vi "Linux Get Time Performance Test.vi"() -> ()   [LabVIEW 2021]
uses:
  <vilib>/Platform/TimedLoop/XDataNode/timing_clust.ctl
  <vilib>/Platform/TimedLoop/XDataNode/nitl_modes.ctl
  <vilib>/Platform/TimedLoop/XDataNode/wakeup.ctl
  <vilib>/Platform/TimedLoop/XDataNode/XDataNode.xnode
  <vilib>/Platform/TimedLoop/XDataNode/XDNodeRunTimeDep.lvlib
  Time_CIF_U.lvlib
panel:
  out "avg Linux Time":dbl
  out "max Linux Time":dbl
  out "avg LV Time":dbl
  out "max LV Time":dbl
  out "pass":bool
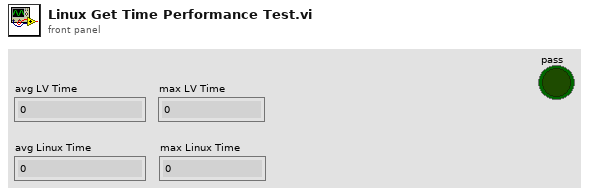
[diagram p1: front panel]
types:
  T1 = typedef "XDNodeRunTimeDep.lvlib/timing_clust.ctl" = cluster{"Expected End [f-1]":u64, "Actual End [f-1]":u64, "Finished Late? [f-1]":bool, "Expected End [i-1]":u64, "Actual End [i-1]":u64, "Finished Late? [i-1]":bool, "Expected Start [i]":u64, "Actual Start [i]":u64, "Expected Start [f]":u64, "Actual Start [f]":u64, "Source Name":string, "Structure Name":string, "Period":i64, "Deadline":i64, "Offset":i64, "Start":i64, "Priority":i32, "Timeout":i32, "Mode":T2, "Wakeup Reason":T3, "Error":errorcluster, "Source Type":string, "Secondary Source Type":string, "Global End Time":u64, "Global Start Time":u64, "Frame Duration":u64, "Iteration Duration":u64, "Assigned CPU":i32, "I/O Scan Engine Mode":u32}
  T2 = typedef "XDNodeRunTimeDep.lvlib/nitl_modes.ctl" = enum32{"No Change", "Process missed periods, maintain original phase", "Discard missed periods, maintain original phase", "Process missed periods, ignore original phase", "Discard missed periods, ignore original phase"}
  T3 = typedef "XDNodeRunTimeDep.lvlib/wakeup.ctl" = enum32{"Normal", "Aborted", "Asynchronous wakeup", "Timing source error", "Timed loop error", "Timeout"}
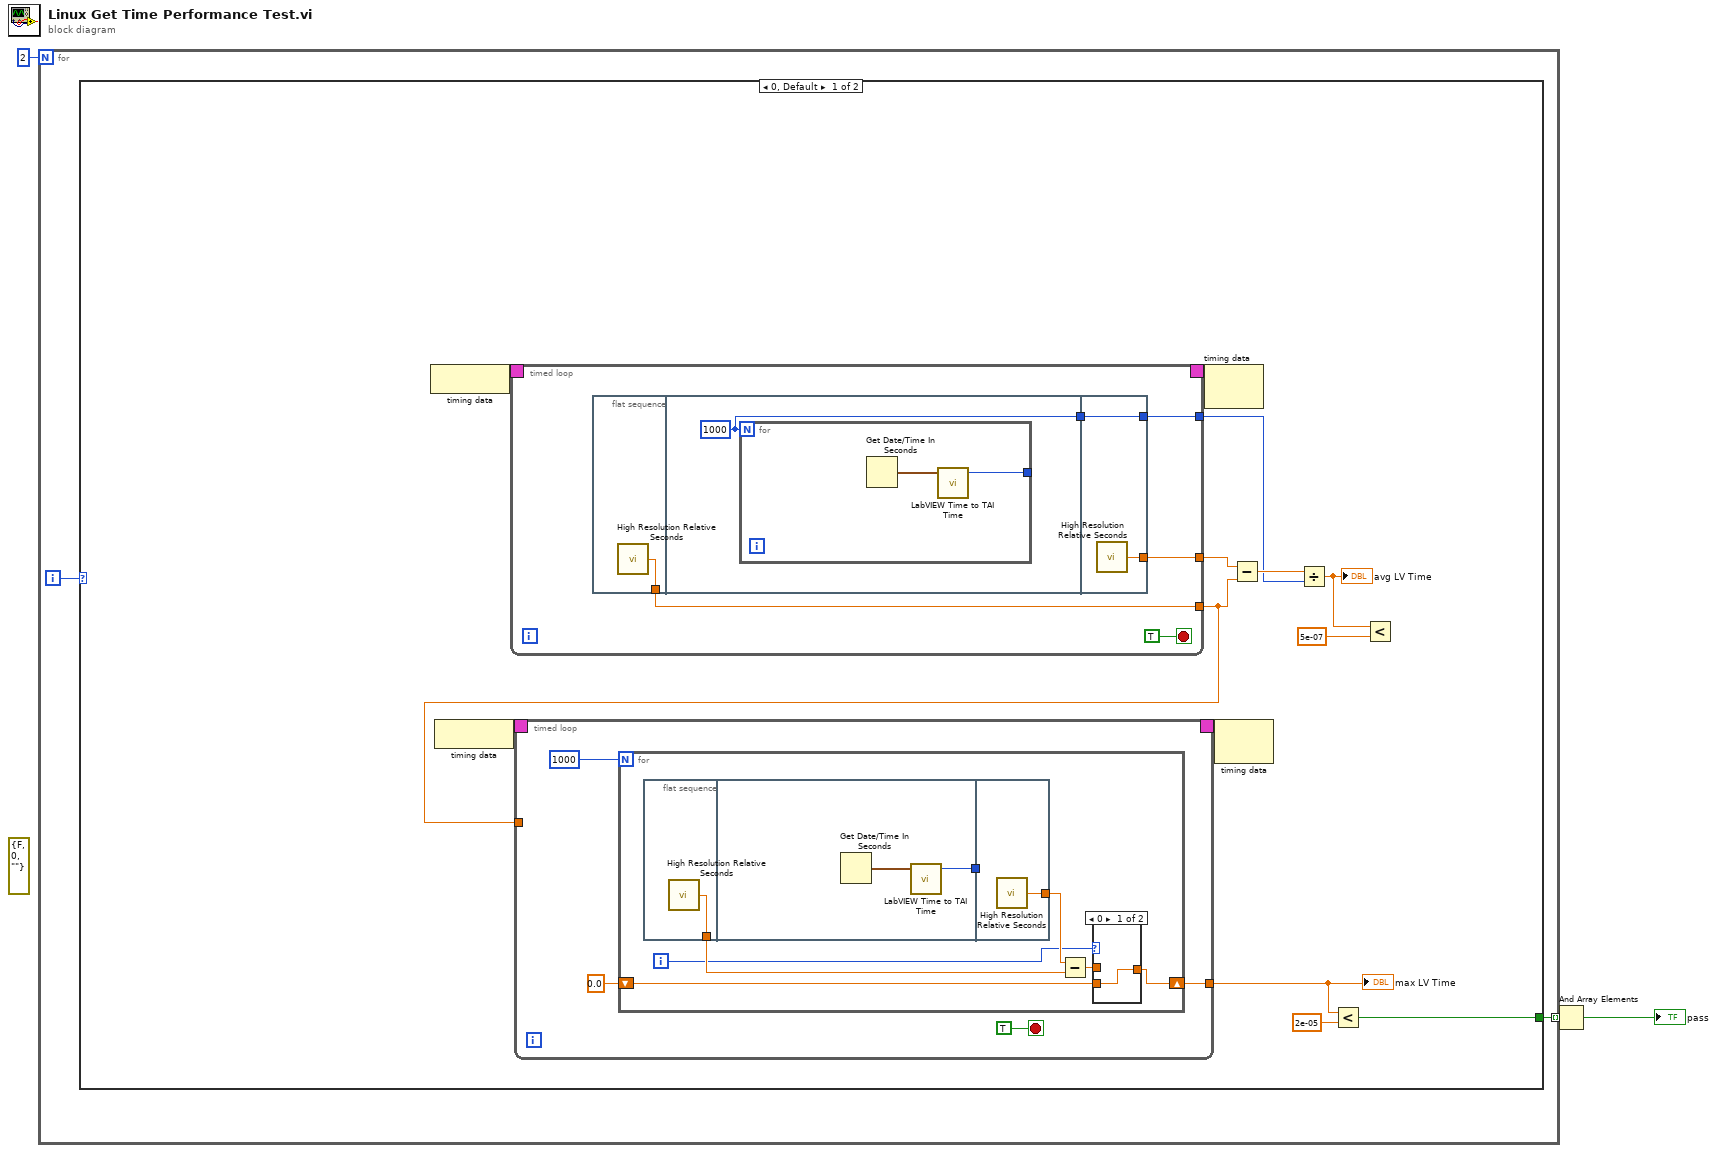
[diagram p0: block diagram]
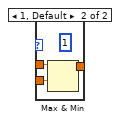
[diagram p2: hidden frame]
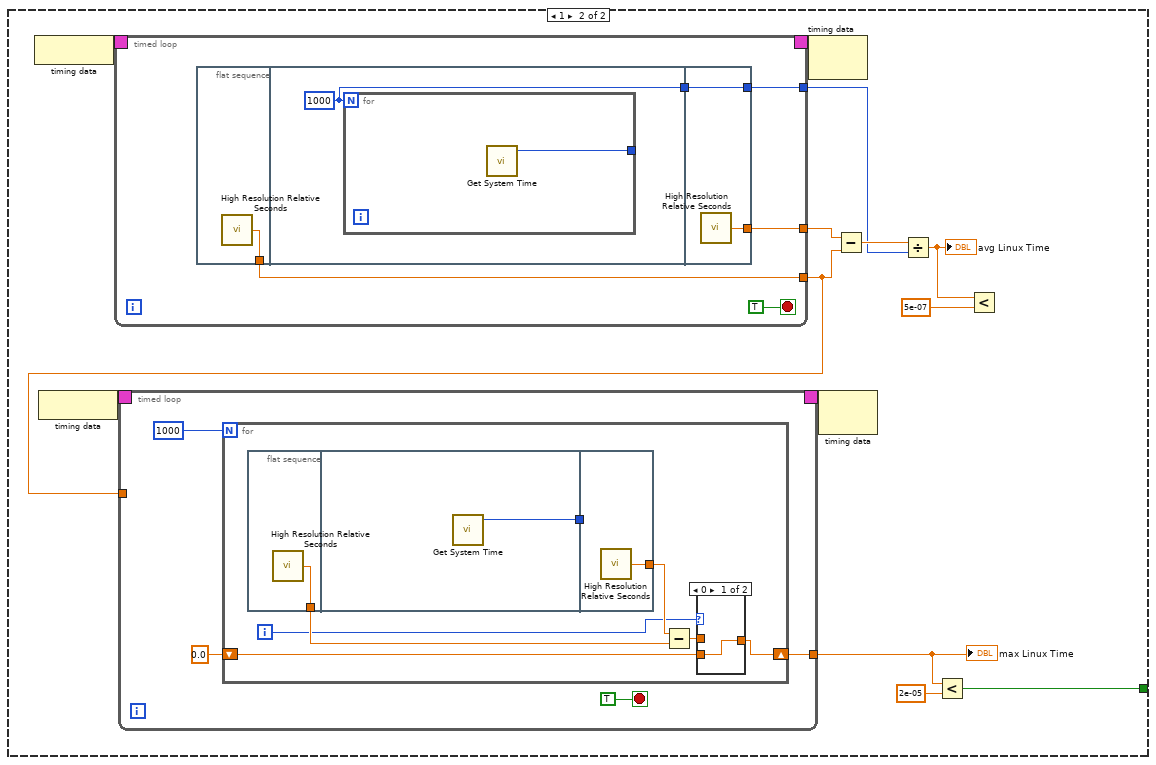
[diagram p3: hidden frame]
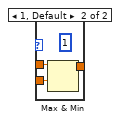
[diagram p4: hidden frame]
diagram:
  (unwired) errorcluster {"status"=FALSE, "code"=0, "source"=""} ("error out")
  n1 = for {
    N: 2 -> [_]
    tunnel: [w5] -> w2 mode=indexing
    i -> [w4]
    n2 = case shown="0, Default" w4 {
      tunnel: [w7 w58] -> w5
      frame 0, Default {
        n3 = node-c288() -> (w18:T1)
        n4 = node-c288() -> (w16:T1)
        n5 = timed-loop {
          timing: w18 -> [_]
          timing-out: [_] -> w17
          tunnel: [w45] -> w14
          tunnel: [w44] -> w6
          tunnel: [w43] -> w12
          stop <- TRUE stop-if-true
          n6 = flat-sequence {
            tunnel: [w47] -> w44
            tunnel: [w48] -> w42
            tunnel: [w52] -> w45
            tunnel: [w51] -> w43
            tunnel: w42 -> [w51]
            frame #0 {
              n7 = call <vilib>:"High Resolution Relative Seconds.vi"() -> ("relative seconds"=w47:dbl)
            }
            frame #1 {
              w48 = 1000
              n8 = for {
                N: w48 -> [_]
                tunnel: [w49] -> _
                n9 = Get Date/Time In Seconds() -> (seconds since 1Jan1904=w50:timestamp)
                n10 = call "LabVIEW Time to TAI Time.vi"("LabVIEW Time (s)"=w50) -> ("TAI Time (ns)"=w49:i64)  [unwired: 4 in]
              }
            }
            frame #2 {
              n11 = call <vilib>:"High Resolution Relative Seconds.vi"() -> ("relative seconds"=w52:dbl)
            }
          }
        }
        n12 = timed-loop {
          timing: w16 -> [_]
          timing-out: [_] -> w15
          tunnel: [w19] -> w9
          tunnel: w6 -> [_]
          stop <- TRUE stop-if-true
          n13 = for {
            N: 1000 -> [_]
            shift-right: [w25] -> w19
            shift-left: 0.0 -> [w26]
            i -> [w24]
            n14 = flat-sequence {
              tunnel: [w34] -> w28
              tunnel: [w35] -> w23
              tunnel: [w37] -> w29
              tunnel: w23 -> [_]
              frame #0 {
                n15 = call <vilib>:"High Resolution Relative Seconds.vi"() -> ("relative seconds"=w34:dbl)
              }
              frame #1 {
                n16 = Get Date/Time In Seconds() -> (seconds since 1Jan1904=w36:timestamp)
                n17 = call "LabVIEW Time to TAI Time.vi"("LabVIEW Time (s)"=w36) -> ("TAI Time (ns)"=w35:i64)  [unwired: 4 in]
              }
              frame #2 {
                n18 = call <vilib>:"High Resolution Relative Seconds.vi"() -> ("relative seconds"=w37:dbl)
              }
            }
            n19 = Subtract(x=w29, y=w28) -> (x-y=w27:dbl)
            n20 = case shown="0" w24 {
              tunnel: w27 -> [_ w33]
              tunnel: w26 -> [w30 w32]
              tunnel: [w30 w31] -> w25
              frame 0 {
              }
              frame 1, Default {
                (unwired) u32 1 ("milliseconds to wait")
                n21 = Max & Min(x=w33, y=w32) -> (max(x,y)=w31:dbl)  [unwired: 1 out]
              }
            }
          }
        }
        "max LV Time" <- w9
        n22 = node-c288(w17) -> ()  [unwired: 1 out]
        n23 = node-c288(w15) -> ()  [unwired: 1 out]
        n24 = Subtract(x=w14, y=w6) -> (x-y=w13:dbl)
        n25 = Divide(x=w13, y=w12) -> (x/y=w11:dbl)
        "avg LV Time" <- w11
        n26 = Less?(x=w9, y=2e-05) -> (x < y?=w7:bool)
        n27 = Less?(x=w11, y=5e-07) -> ()  [unwired: 1 out]
      }
      frame 1 {
        n28 = node-c288() -> (w69:T1)
        n29 = node-c288() -> (w67:T1)
        n30 = timed-loop {
          timing: w69 -> [_]
          timing-out: [_] -> w68
          tunnel: [w95] -> w65
          tunnel: [w94] -> w57
          tunnel: [w93] -> w63
          stop <- TRUE stop-if-true
          n31 = flat-sequence {
            tunnel: [w97] -> w94
            tunnel: [w98] -> w92
            tunnel: [w101] -> w95
            tunnel: [w100] -> w93
            tunnel: w92 -> [w100]
            frame #0 {
              n32 = call <vilib>:"High Resolution Relative Seconds.vi"() -> ("relative seconds"=w97:dbl)
            }
            frame #1 {
              w98 = 1000
              n33 = for {
                N: w98 -> [_]
                tunnel: [w99] -> _
                n34 = call "Get System Time.vi"() -> ("Time (ns)"=w99:i64)  [unwired: 5 in]
              }
            }
            frame #2 {
              n35 = call <vilib>:"High Resolution Relative Seconds.vi"() -> ("relative seconds"=w101:dbl)
            }
          }
        }
        n36 = timed-loop {
          timing: w67 -> [_]
          timing-out: [_] -> w66
          tunnel: [w70] -> w60
          tunnel: w57 -> [_]
          stop <- TRUE stop-if-true
          n37 = for {
            N: 1000 -> [_]
            shift-right: [w76] -> w70
            shift-left: 0.0 -> [w77]
            i -> [w75]
            n38 = flat-sequence {
              tunnel: [w85] -> w79
              tunnel: [w86] -> w74
              tunnel: [w87] -> w80
              tunnel: w74 -> [_]
              frame #0 {
                n39 = call <vilib>:"High Resolution Relative Seconds.vi"() -> ("relative seconds"=w85:dbl)
              }
              frame #1 {
                n40 = call "Get System Time.vi"() -> ("Time (ns)"=w86:i64)  [unwired: 5 in]
              }
              frame #2 {
                n41 = call <vilib>:"High Resolution Relative Seconds.vi"() -> ("relative seconds"=w87:dbl)
              }
            }
            n42 = Subtract(x=w80, y=w79) -> (x-y=w78:dbl)
            n43 = case shown="0" w75 {
              tunnel: w78 -> [_ w84]
              tunnel: w77 -> [w81 w83]
              tunnel: [w81 w82] -> w76
              frame 0 {
              }
              frame 1, Default {
                (unwired) u32 1 ("milliseconds to wait")
                n44 = Max & Min(x=w84, y=w83) -> (max(x,y)=w82:dbl)  [unwired: 1 out]
              }
            }
          }
        }
        "max Linux Time" <- w60
        n45 = node-c288(w68) -> ()  [unwired: 1 out]
        n46 = node-c288(w66) -> ()  [unwired: 1 out]
        n47 = Subtract(x=w65, y=w57) -> (x-y=w64:dbl)
        n48 = Divide(x=w64, y=w63) -> (x/y=w62:dbl)
        "avg Linux Time" <- w62
        n49 = Less?(x=w60, y=2e-05) -> (x < y?=w58:bool)
        n50 = Less?(x=w62, y=5e-07) -> ()  [unwired: 1 out]
      }
    }
  }
  n51 = And Array Elements(Boolean array=w2) -> (logical AND=→"pass":bool)
